vi "ParameterCfgSave.vi"(0 "config_values":string[][](array[string]), 1 "section":string, 2 "appended path":path) -> ()   [LabVIEW 2019]
uses:
  <vilib>/Utility/config.llb/Write Key (Double).vi
  <vilib>/Utility/config.llb/Write Key (String).vi
  <vilib>/Utility/config.llb/NI_LVConfig.lvlib
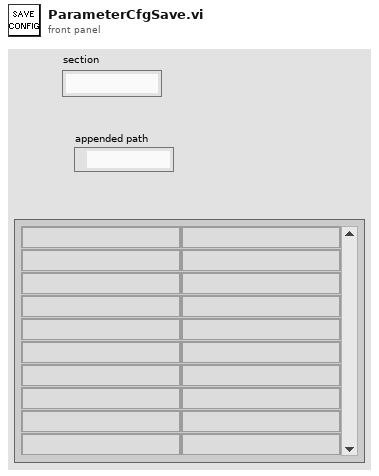
[diagram p1: front panel]
types:
  T1 = typedef "NI_LVConfig.lvlib/Config Data RefNum.ctl" = refnum<k1>
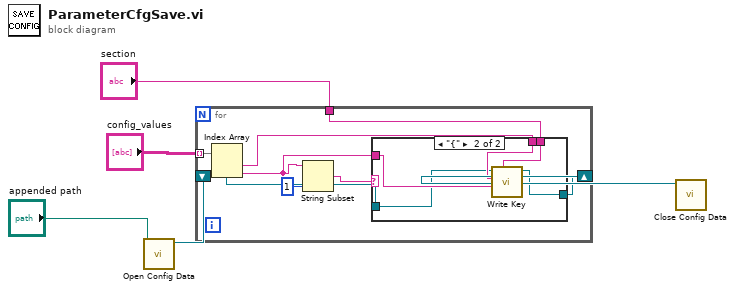
[diagram p0: block diagram]
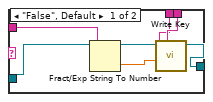
[diagram p2: hidden frame]
diagram:
  n1 = call <vilib>:"Open Config Data.vi"("configuration file path"="appended path") -> ("refnum"=w4:T1)  [unwired: 8 in, 2 out]
  n2 = for {
    tunnel: "config_values" -> [w11] mode=indexing
    shift-right: [w12] -> w2
    shift-left: w4 -> [w13]
    tunnel: "section" -> [w10]
    n3 = Index Array(array=w11) -> (element #1=w9:string, element #2=w6:string)  [unwired: 2 in]
    n4 = String Subset(string=w6, length (rest)=1 ("length (rest)")) -> (substring=w7:string)  [unwired: 1 in]
    n5 = case shown="\"{\"" w7 {
      tunnel: w13 -> [w19 w20]
      tunnel: [w15 w21] -> w12
      tunnel: w10 -> [w17 w22]
      tunnel: w9 -> [w16 w23]
      tunnel: w6 -> [w14 w24]
      frame "False", Default {
        n6 = Fract/Exp String To Number(string=w14) -> (number=w18:dbl)  [unwired: 3 in, 1 out]
        n7 = call-poly <vilib>:"Write Key.vi"("section"=w17, "value"=w18, "key"=w16, "refnum"=w19) -> ("refnum out"=w15:T1)  [unwired: 5 in, 2 out]
      }
      frame "{" {
        n8 = call-poly <vilib>:"Write Key.vi"("section"=w22, "value"=w24, "key"=w23, "refnum"=w20) -> ("refnum out"=w21:T1)  [unwired: 5 in, 2 out]
      }
    }
  }
  n9 = call <vilib>:"Close Config Data.vi"("refnum"=w2) -> ()  [unwired: 9 in, 2 out]
